vi "1762SweepTrigWvfmBuilder.vi"(1 "Sweep Trigger":digitalwaveform(waveform)={"t0"=timestamp(0 s since 1904-01-01), "dt"=0.0, "Y"={"transitions"=[], "data"=[]}, "error"={"status"=FALSE, "code"=37421928, "source"=""}}, 2 "pockel":digitalwaveform(waveform)={"t0"=timestamp(0 s since 1904-01-01), "dt"=0.0, "Y"={"transitions"=[], "data"=[]}, "error"={"status"=FALSE, "code"=37421928, "source"=""}}, 3 "614":digitalwaveform(waveform)={"t0"=timestamp(0 s since 1904-01-01), "dt"=0.0, "Y"={"transitions"=[], "data"=[]}, "error"={"status"=FALSE, "code"=37421928, "source"=""}}, 4 "1762":digitalwaveform(waveform)={"t0"=timestamp(0 s since 1904-01-01), "dt"=0.0, "Y"={"transitions"=[], "data"=[]}, "error"={"status"=FALSE, "code"=37421928, "source"=""}}, 5 "650":digitalwaveform(waveform)={"t0"=timestamp(0 s since 1904-01-01), "dt"=0.0, "Y"={"transitions"=[], "data"=[]}, "error"={"status"=FALSE, "code"=37421928, "source"=""}}, 6 "493":digitalwaveform(waveform)={"t0"=timestamp(0 s since 1904-01-01), "dt"=0.0, "Y"={"transitions"=[], "data"=[]}, "error"={"status"=FALSE, "code"=37421928, "source"=""}}) -> (0 "out":digitalwaveform(waveform)={"t0"=timestamp(0 s since 1904-01-01), "dt"=0.0, "Y"={"transitions"=[], "data"=[]}, "error"={"status"=FALSE, "code"=37421928, "source"=""}})   [LabVIEW 2012]
uses:
  <vilib>/Waveform/DWDTOps.llb/DWDT Append Digital Signals.vi
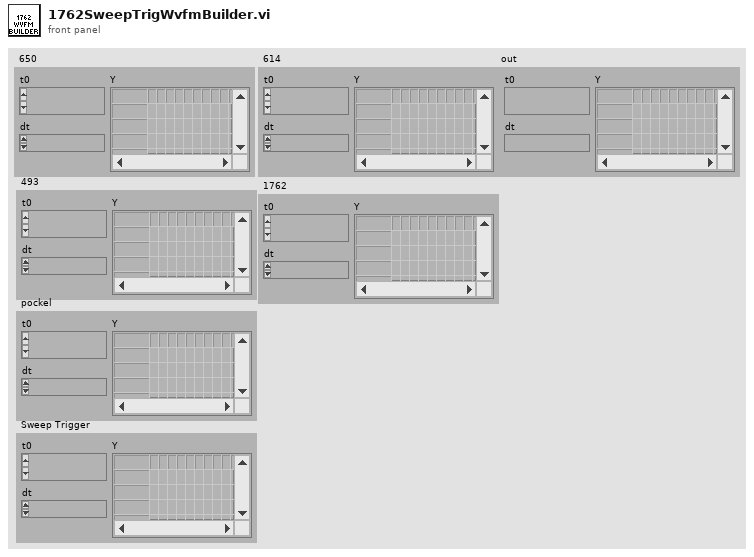
[diagram p1: front panel]
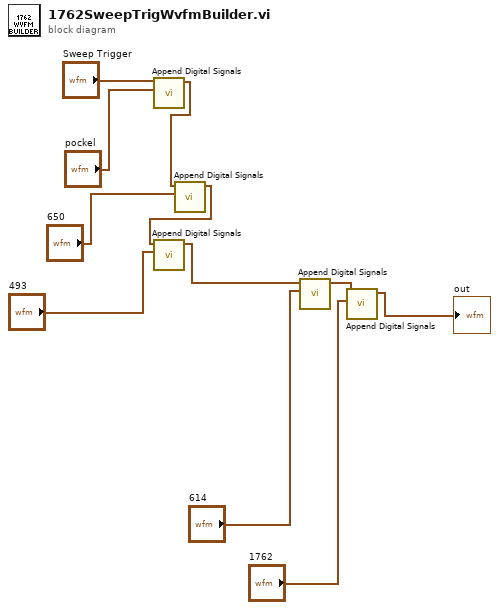
[diagram p0: block diagram]
diagram:
  n1 = call-poly <vilib>:"Append Digital Signals.vi"("digital waveform (low bits)"="pockel", "digital waveform (high bits)"="Sweep Trigger") -> ("digital waveform out"=w1:digitalwaveform)  [unwired: 8 in, 1 out]
  n2 = call-poly <vilib>:"Append Digital Signals.vi"("digital waveform (low bits)"="650", "digital waveform (high bits)"=w1) -> ("digital waveform out"=w4:digitalwaveform)  [unwired: 8 in, 1 out]
  n3 = call-poly <vilib>:"Append Digital Signals.vi"("digital waveform (low bits)"="493", "digital waveform (high bits)"=w4) -> ("digital waveform out"=w7:digitalwaveform)  [unwired: 8 in, 1 out]
  n4 = call-poly <vilib>:"Append Digital Signals.vi"("digital waveform (low bits)"="614", "digital waveform (high bits)"=w7) -> ("digital waveform out"=w10:digitalwaveform)  [unwired: 8 in, 1 out]
  n5 = call-poly <vilib>:"Append Digital Signals.vi"("digital waveform (low bits)"="1762", "digital waveform (high bits)"=w10) -> ("digital waveform out"=→"out":digitalwaveform)  [unwired: 8 in, 1 out]
